vi "Auton File Control.vi"(10 "Manip D-Pad":T1, 11 "Manip Button":T2) -> ()   [LabVIEW 2015]
uses:
  Common Code/Gamepads/Button Cluster.ctl
  Common Code/Gamepads/D-Pad.ctl
  Common Code/Change Detect Boolean.vi
  Common Code/Change Detect Int.vi
  Robot Global Data.vi
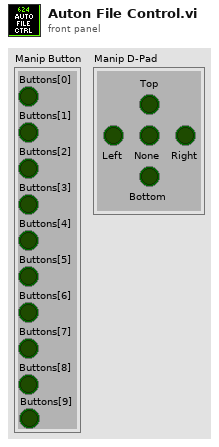
[diagram p1: front panel]
types:
  T1 = typedef "D-Pad.ctl" = cluster{"Top":bool, "Bottom":bool, "None":bool, "Right":bool, "Left":bool}
  T2 = typedef "Button Cluster.ctl" = cluster{"Buttons[0]":bool, "Buttons[1]":bool, "Buttons[2]":bool, "Buttons[3]":bool, "Buttons[4]":bool, "Buttons[5]":bool, "Buttons[6]":bool, "Buttons[7]":bool, "Buttons[8]":bool, "Buttons[9]":bool}
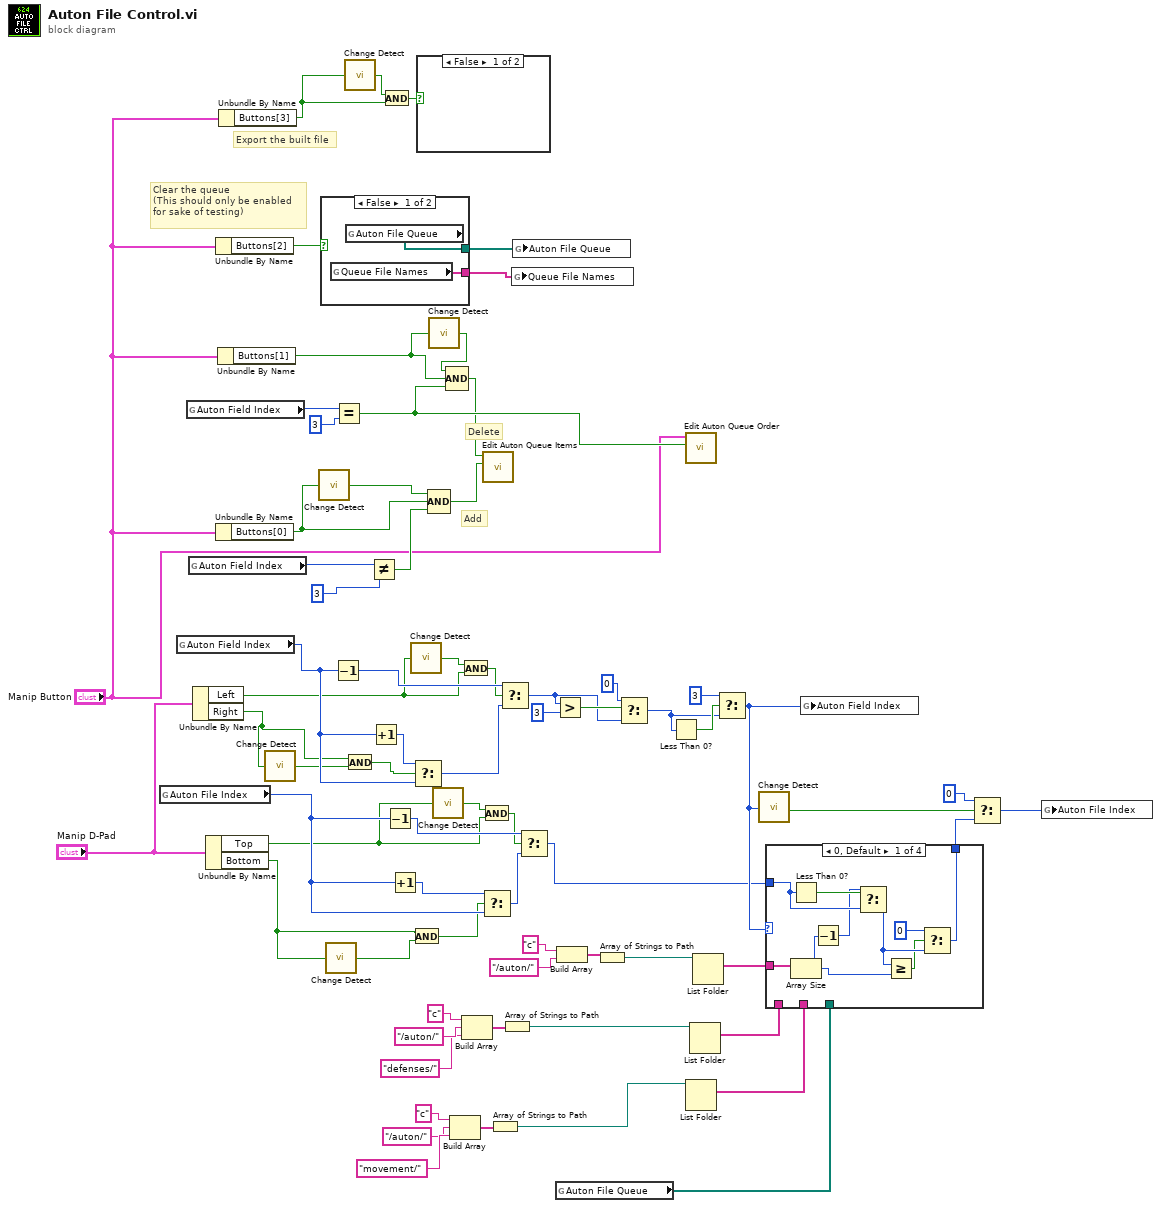
[diagram p0: block diagram]
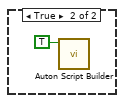
[diagram p2: hidden frame]
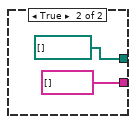
[diagram p3: hidden frame]
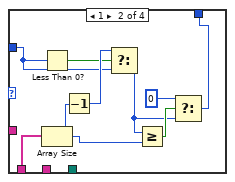
[diagram p4: hidden frame]
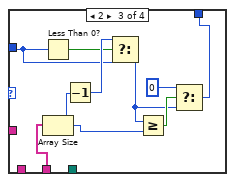
[diagram p5: hidden frame]
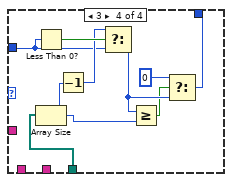
[diagram p6: hidden frame]
diagram:
  # "Clear the queue\n(This should only be enabled\nfor sake of testing)"
  # "Export the built file"
  # "Delete"
  # "Add"
  n1 = global read "Robot Global Data.vi" "Auton File Index"() -> (w57:i32)
  n2 = global read "Robot Global Data.vi" "Auton Field Index"() -> (w69:i32)
  n3 = global read "Robot Global Data.vi" "Auton Field Index"() -> (w46:i32)
  n4 = global read "Robot Global Data.vi" "Auton Field Index"() -> (w43:i32)
  n5 = Unbundle By Name("Manip D-Pad") -> ("Left"=w12:bool, "Right"=w7:bool)
  n6 = Unbundle By Name("Manip D-Pad") -> ("Top"=w11:bool, "Bottom"=w10:bool)
  n7 = Unbundle By Name("Manip Button") -> ("Buttons[2]"=w14:bool)
  n8 = Unbundle By Name("Manip Button") -> ("Buttons[0]"=w9:bool)
  n9 = Unbundle By Name("Manip Button") -> ("Buttons[1]"=w8:bool)
  n10 = Unbundle By Name("Manip Button") -> ("Buttons[3]"=w3:bool)
  n11 = call-poly "Change Detect.vi"("In"=w7) -> ("Changed?"=w20:bool)
  n12 = call-poly "Change Detect.vi"("In"=w9) -> ("Changed?"=w28:bool)
  n13 = case shown="False" w14 {
    tunnel: [w73 path[] [] ("Auton File Queue")] -> w13
    tunnel: [w72 string[] []] -> w1
    frame False {
      n14 = global read "Robot Global Data.vi" "Queue File Names"() -> (w72:string[])
      n15 = global read "Robot Global Data.vi" "Auton File Queue"() -> (w73:path[])
    }
    frame True {
    }
  }
  n16 = call-poly "Change Detect.vi"("In"=w10) -> ("Changed?"=w16:bool)
  n17 = Decrement(x=w69) -> (x-1=w71:i32)
  n18 = Equal?(x=w46, y=3) -> (x = y?=w25:bool)
  n19 = call-poly "Change Detect.vi"("In"=w3) -> ("Changed?"=w4:bool)
  n20 = And(x=w7, y=w20) -> (x .and. y?=w19:bool)
  n21 = Not Equal?(x=w43, y=3) -> (x != y?=w27:bool)
  n22 = Increment(x=w69) -> (x+1=w70:i32)
  n23 = And(x=w4, y=w3) -> (x .and. y?=w5:bool)
  n24 = Decrement(x=w57) -> (x-1=w58:i32)
  n25 = Increment(x=w57) -> (x+1=w59:i32)
  n26 = call-poly "Change Detect.vi"("In"=w12) -> ("Changed?"=w22:bool)
  n27 = And(x=w10, y=w16) -> (x .and. y?=w15:bool)
  n28 = Select(t=w70, s=w19, f=w69) -> (s? t:f=w68:i32)
  n29 = case shown="False" w5 {
    frame False {
    }
    frame True {
      n30 = call "Auton Script Builder.vi"("Export?"=TRUE) -> ()  [unwired: 11 in]
    }
  }
  n31 = Compound Arithmetic op=AND(w28, w9, w27) -> (w26:bool)
  n32 = call-poly "Change Detect.vi"("In"=w8) -> ("Changed?"=w24:bool)
  n33 = call-poly "Change Detect.vi"("In"=w11) -> ("Changed?"=w18:bool)
  n34 = Compound Arithmetic op=AND(w24, w8, w25) -> (w23:bool)
  n35 = Build Array("c", "/auton/", "movement/" ("element")) -> (w37:string[])
  n36 = And(x=w22, y=w12) -> (x .and. y?=w21:bool)
  n37 = Build Array("c", "/auton/", "defenses/" ("element")) -> (w41:string[])
  n38 = And(x=w18, y=w11) -> (x .and. y?=w17:bool)
  n39 = Select(t=w59, s=w15, f=w57) -> (s? t:f=w60:i32)
  n40 = call "Edit Auton Queue Items.vi"("Add?"=w26, "Delete?"=w23) -> ()  [unwired: 10 in]
  n41 = Array of Strings to Path(0:w37) -> (2:w35:path)  [unwired: 1 in]
  n42 = Select(t=w71, s=w21, f=w68) -> (s? t:f=w65:i32)
  n43 = Array of Strings to Path(0:w41) -> (2:w39:path)  [unwired: 1 in]
  n44 = global write "Robot Global Data.vi" "Queue File Names"(w1) -> ()
  n45 = global write "Robot Global Data.vi" "Auton File Queue"(w13) -> ()
  n46 = Select(t=w58, s=w17, f=w60) -> (s? t:f=w55:i32)
  n47 = Greater?(x=w65, y=3) -> (0:w66:bool)
  n48 = global read "Robot Global Data.vi" "Auton File Queue"() -> (w51:path[])
  n49 = Build Array("c", "/auton/") -> (w31:string[])
  n50 = Array of Strings to Path(0:w31) -> (2:w29:path)  [unwired: 1 in]
  n51 = Select(t=0, s=w66, f=w65) -> (s? t:f=w62:i32)
  n52 = Less Than 0?(x=w62) -> (x < 0?=w63:bool)
  n53 = call "Edit Auton Queue Order.vi"("Boolean"=w25, "Manip Button"="Manip Button") -> ()  [unwired: 10 in]
  n54 = List Folder(path=w35) -> (filenames=w52:string[])  [unwired: 3 in, 3 out]
  n55 = List Folder(path=w39) -> (filenames=w53:string[])  [unwired: 3 in, 3 out]
  n56 = List Folder(path=w29) -> (filenames=w54:string[])  [unwired: 3 in, 3 out]
  n57 = Select(t=3, s=w63, f=w62) -> (s? t:f=w56:i32)
  n58 = call-poly "Change Detect.vi"("In"=w56) -> ("Changed?"=w50:bool)
  n59 = case shown="0, Default" w56 {
    tunnel: w55 -> [w83 w87 w96 w105]
    tunnel: w54 -> [w85 _ _ _]
    tunnel: w53 -> [_ w88 _ _]
    tunnel: w52 -> [_ _ w97 _]
    tunnel: w51 -> [_ _ _ w104]
    tunnel: [w77 w86 w95 w106] -> w49
    frame 0, Default {
      n60 = Less Than 0?(x=w83) -> (x < 0?=w84:bool)
      n61 = Array Size(array=w85) -> (size(s)=w80:i32)
      n62 = Decrement(x=w80) -> (x-1=w82:i32)
      n63 = Select(t=w82, s=w84, f=w83) -> (s? t:f=w81:i32)
      n64 = Greater Or Equal?(x=w81, y=w80) -> (x >= y?=w79:bool)
      n65 = Select(t=0, s=w79, f=w81) -> (s? t:f=w77:i32)
    }
    frame 1 {
      n66 = Less Than 0?(x=w87) -> (x < 0?=w89:bool)
      n67 = Array Size(array=w88) -> (size(s)=w92:i32)
      n68 = Decrement(x=w92) -> (x-1=w90:i32)
      n69 = Select(t=w90, s=w89, f=w87) -> (s? t:f=w91:i32)
      n70 = Greater Or Equal?(x=w91, y=w92) -> (x >= y?=w93:bool)
      n71 = Select(t=0, s=w93, f=w91) -> (s? t:f=w86:i32)
    }
    frame 2 {
      n72 = Less Than 0?(x=w96) -> (x < 0?=w98:bool)
      n73 = Array Size(array=w97) -> (size(s)=w101:i32)
      n74 = Decrement(x=w101) -> (x-1=w99:i32)
      n75 = Select(t=w99, s=w98, f=w96) -> (s? t:f=w100:i32)
      n76 = Greater Or Equal?(x=w100, y=w101) -> (x >= y?=w102:bool)
      n77 = Select(t=0, s=w102, f=w100) -> (s? t:f=w95:i32)
    }
    frame 3 {
      n78 = Less Than 0?(x=w105) -> (x < 0?=w112:bool)
      n79 = Array Size(array=w104) -> (size(s)=w109:i32)
      n80 = Decrement(x=w109) -> (x-1=w111:i32)
      n81 = Select(t=w111, s=w112, f=w105) -> (s? t:f=w110:i32)
      n82 = Greater Or Equal?(x=w110, y=w109) -> (x >= y?=w108:bool)
      n83 = Select(t=0, s=w108, f=w110) -> (s? t:f=w106:i32)
    }
  }
  n84 = global write "Robot Global Data.vi" "Auton Field Index"(w56) -> ()
  n85 = Select(t=0, s=w50, f=w49) -> (s? t:f=w47:i32)
  n86 = global write "Robot Global Data.vi" "Auton File Index"(w47) -> ()
